vi "GetAttributeViString_Advanced.vi"(7 "AttributeValueBufferSize":i32=256 caption="AttributeValueBufferSize (256)", 8 "error in (no error)":errorcluster {"code" format="%.0x"}, 9 "AttributeID":u32(ring)=1950012 items=["IVILXISYNC_ARM_SOURCE_EVENTID"=1950012, "IVILXISYNC_ARM_SOURCE_FILTER"=1950013, "IVILXISYNC_EVENT_DESTINATION_PATH"=1950029, "IVILXISYNC_EVENT_SOURCE"=1950032, "IVILXISYNC_TRIGGER_SOURCE"=1950022, "IVILXISYNC_TRIGGER_SOURCE_EVENTID"=1950026, "IVILXISYNC_TRIGGER_SOURCE_FILTER"=1950027, "LOGICAL_NAME"=1050305, "MARKER_TRACE"=1250209, "SPECIFIC_DRIVER_DESCRIPTION"=1050514, "SPECIFIC_DRIVER_REVISION"=1050551, "SPECIFIC_DRIVER_VENDOR"=1050513, "STATETRIGGER_EVENT_ID"=1150161, "STATETRIGGER_FILTER"=1150162, "STATETRIGGER_STATE_LOCATION"=1150163, "SUPPORTED_INSTRUMENT_MODELS"=1050327, "SYSTEM_DATE"=1150172, "SYSTEM_SERIAL_NUMBER"=1150173, "SYSTEM_TIME"=1150174, "TEXT"=1150431], 10 "RepCapIdentifier":string, 11 "instrument handle":refnum<k15>) -> (0 "error out":errorcluster {"code" format="%.0x"}, 2 "AttributeValue":string, 3 "instrument handle out":refnum<k15>)   [LabVIEW 2009, in "Keysight XSAn.lvlib"]
doc: "Gets a String attribute from the instrument driver.\nThe following Attributes are supported:\n\nIVILXISYNC_ARM_SOURCE_EVENTID\nIVILXISYNC_ARM_SOURCE_FILTER\nIVILXISYNC_EVENT_DESTINATION_PATH\nIVILXISYNC_EVENT_SOURCE\nIVILXISYNC_TRIGGER_SOURCE\nIVILXISYNC_TRIGGER_SOURCE_EVENTID\nIVILXISYNC_TRIGGER_SOURCE_FILTER\nLOGICAL_NAME\nMARKER_TRACE\nSPECIFIC_DRIVER_DESCRIPTION\nSPECIFIC_DRIVER_REVISION\nSPECIFIC_DRIVER_VENDOR\nSTATETRIGGER_EVENT_ID\nSTATETRIGGER_FILTER\nSTATETRIGGER_STATE_LOCATION\nSUPPORTED_INSTRUMENT_MODELS\nSYSTEM_DATE\nSYSTEM_SERIAL_NUMBER\nSYSTEM_TIME\nTEXT"
uses:
  <instrlib>/Keysight XSAn/Keysight XSAn.lvlib
  AgXSAn.dll
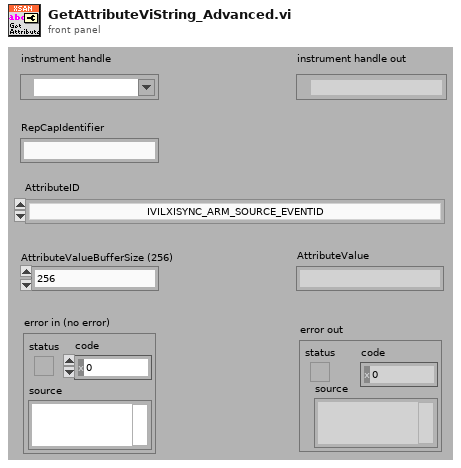
[diagram p1: front panel]
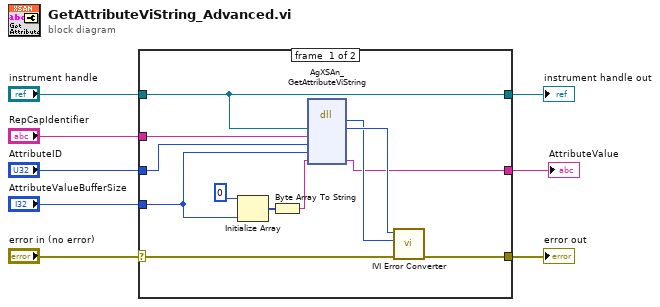
[diagram p0: block diagram]
diagram:
  n1 = case shown="No Error" "error in (no error)" {
    selector: "error in (no error)" -> [w18 w22]
    tunnel: [w17 w22] -> w8
    tunnel: "instrument handle" -> [w10 w21]
    tunnel: "RepCapIdentifier" -> [w16 _]
    tunnel: "AttributeID" -> [w15 _]
    tunnel: "AttributeValueBufferSize" -> [w9 _]
    tunnel: [w11 _] -> w2
    tunnel: [w10 w21] -> w1
    frame #0 {
      n2 = Initialize Array(u8 0 ("element"), w9) -> (w13:u8[])
      n3 = Byte Array To String(unsigned byte array=w13) -> (string=w14:string)
      n4 = dll-call lib="AgXSAn**.dll" fn="AgXSAn_GetAttributeViString"("Vi"=w10, "RepCapIdentifier"=w16, "AttributeID"=w15, "AttributeValueBufferSize"=w9, "AttributeValue"=w14) -> ("return type"=w19:i32, "Vi"=w20:u32, "AttributeValue"=w11:string)  [unwired: 6 in, 2 out]
      n5 = call <instrlib>:"IVI Error Converter.vi"("error in (no error)"=w18, "IVI error code (0)"=w19, "instrument handle"=w20) -> ("error out"=w17:errorcluster)  [unwired: 7 in, 1 out]
    }
    frame #1 {
    }
  }
  "error out" <- w8
  "instrument handle out" <- w1
  "AttributeValue" <- w2
